vi "StoreSystemConfig.vi"(4 "Version":string(combo), 5 "StoreConfigCommand":T1, 6 "error in":errorcluster, 8 "Table Control":string[](array[string]), 9 "Strings []":string[](array[string])) -> (0 "error out":errorcluster, 2 "All Data":string[][](array[string]), 3 "AvailableVersions":string[](array[string]))   [LabVIEW 2023]
doc: "*-----------------------------------------------------\n* Author: SWatts\n*\n* VI Description: Stores system data to config dB\n* \n*\n* Error handling: All errors passed out\n*\n* Pre-condition: \n*\n* Post-condition: None\n*\n* Revision History:\n*\n* Rev Date Author Description \n* 01 30/04/2014 SWatts First issue\n*\n*-----------------------------------------------------"
uses:
  ConfigCommand.ctl
  System Config Data Manager Parameter.ctl
  StoreCommand.ctl
panel:
  in  "SysParameter":T2
  # "Input"
  # "Output"
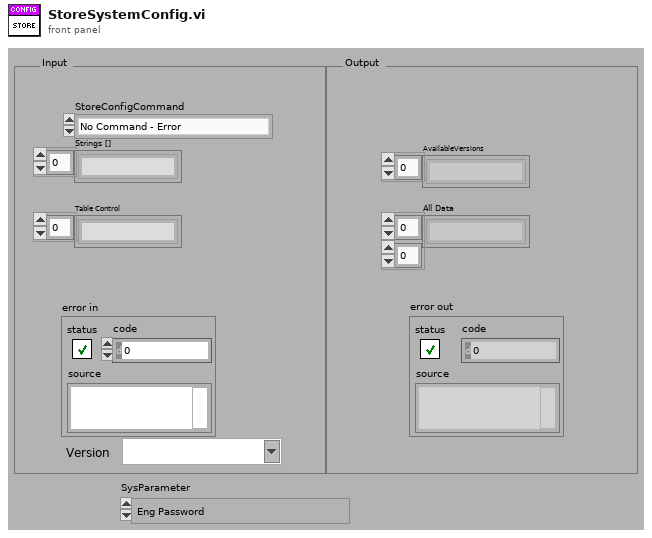
[diagram p1: front panel]
types:
  T1 = typedef "StoreCommand.ctl" = enum16{"No Command - Error", "Store New Version From Inputs", "Update From Input", "Store from dB"}
  T2 = typedef "System Config Data Manager Parameter.ctl" = enum16{"Eng Password", "DSN Connection", "User Password", "RunStatus", "InitialDataPath", "helpFilePath", "ErrorFilepath", "DatalogPath", "Hello"}
  T3 = typedef "ConfigCommand.ctl" = enum16{"No Command - Error", "Initialise Config SQLite", "Save Config", "Get Key", "Set Key", "Update Key", "Get Latest Config Data", "Get Config Data for Version", "Get Default Config Data"}
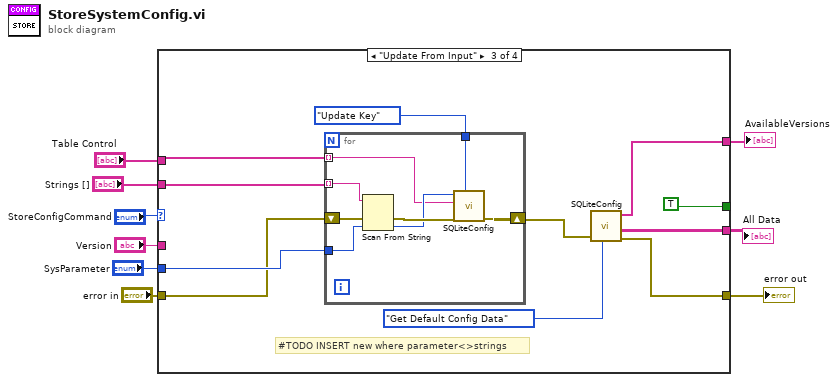
[diagram p0: block diagram]
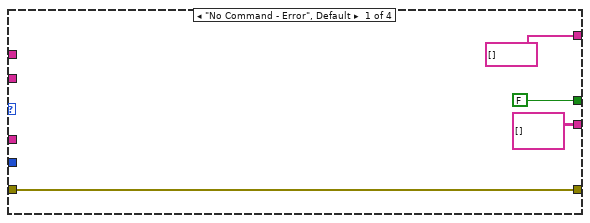
[diagram p2: hidden frame]
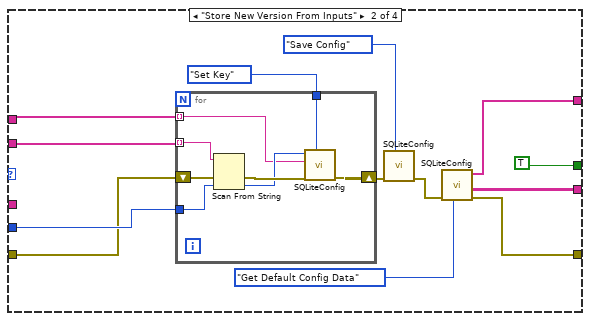
[diagram p3: hidden frame]
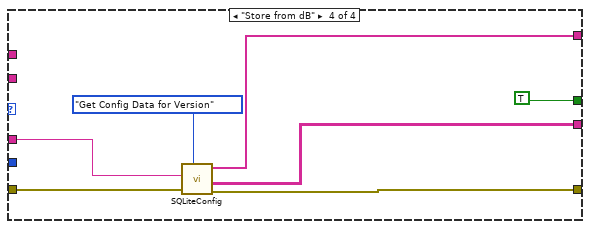
[diagram p4: hidden frame]
diagram:
  n1 = case shown="\"Update From Input\"" "StoreConfigCommand" {
    tunnel: "error in" -> [w12 w16 w38 w59]
    tunnel: [w12 w21 w42 w57] -> w1
    tunnel: [FALSE TRUE TRUE TRUE] -> _
    tunnel: "Version" -> [_ _ _ w58]
    tunnel: "Table Control" -> [_ w15 w37 _]
    tunnel: "Strings []" -> [_ w14 w36 _]
    tunnel: "SysParameter" -> [_ w22 w43 _]
    tunnel: [string[] [] ("Table Control") w20 w41 w54] -> w3
    tunnel: [string[][] [] ("All Data") w19 w40 w55] -> w2
    frame "No Command - Error", Default {
    }
    frame "Store New Version From Inputs" {
      n2 = for {
        tunnel: w15 -> [w28] mode=indexing
        tunnel: w14 -> [w33] mode=indexing
        tunnel: w22 -> [w34]
        shift-right: [w31] -> w23
        shift-left: w16 -> [w32]
        tunnel: ConfigCommand."Set Key" ("ConfigCommand") -> [w27]
        n3 = Scan From String(input string=w33, error in=w32, default 1=w34) -> (error out=w30:errorcluster, output 1=w29:T2)  [unwired: 2 in, 2 out]
        n4 = call "SQLiteConfig.vi"("ConfigCommand"=w27, "error in (no error)"=w30, "KeyDataIn"=w28, "Parameter"=w29) -> ("error out"=w31:errorcluster)  [unwired: 1 in, 3 out]
      }
      n5 = call "SQLiteConfig.vi"("ConfigCommand"=ConfigCommand."Save Config", "error in (no error)"=w23) -> ("error out"=w24:errorcluster)  [unwired: 3 in, 3 out]
      n6 = call "SQLiteConfig.vi"("ConfigCommand"=ConfigCommand."Get Default Config Data", "error in (no error)"=w24) -> ("error out"=w21:errorcluster, "All Data"=w19:string[][], "AvailableVersions"=w20:string[])  [unwired: 3 in, 1 out]
    }
    frame "Update From Input" {
      # "#TODO INSERT new where parameter<>strings"
      n7 = for {
        tunnel: w37 -> [w47] mode=indexing
        tunnel: w36 -> [w52] mode=indexing
        tunnel: w43 -> [w53]
        shift-right: [w50] -> w35
        shift-left: w38 -> [w51]
        tunnel: ConfigCommand."Update Key" ("ConfigCommand") -> [w46]
        n8 = Scan From String(input string=w52, error in=w51, default 1=w53) -> (error out=w49:errorcluster, output 1=w48:T2)  [unwired: 2 in, 2 out]
        n9 = call "SQLiteConfig.vi"("ConfigCommand"=w46, "error in (no error)"=w49, "KeyDataIn"=w47, "Parameter"=w48) -> ("error out"=w50:errorcluster)  [unwired: 1 in, 3 out]
      }
      n10 = call "SQLiteConfig.vi"("ConfigCommand"=ConfigCommand."Get Default Config Data", "error in (no error)"=w35) -> ("error out"=w42:errorcluster, "All Data"=w40:string[][], "AvailableVersions"=w41:string[])  [unwired: 3 in, 1 out]
    }
    frame "Store from dB" {
      n11 = call "SQLiteConfig.vi"("ConfigCommand"=ConfigCommand."Get Config Data for Version", "error in (no error)"=w59, "KeyDataIn"=w58) -> ("error out"=w57:errorcluster, "All Data"=w55:string[][], "AvailableVersions"=w54:string[])  [unwired: 2 in, 1 out]
    }
  }
  "error out" <- w1
  "All Data" <- w2
  "AvailableVersions" <- w3
